vi "playsound.vi"(11 "Sound File Path":path=path "../support/sample.wav") -> ()   [LabVIEW 2014]
uses:
  <vilib>/sound2/lvsound2.llb/Sampling Mode.ctl
  <vilib>/sound2/lvsound2.llb/Sound File Info (path).vi
  <vilib>/sound2/lvsound2.llb/Sound File Read Open.vi
  <vilib>/sound2/lvsound2.llb/Sound File Read (DBL).vi
  <vilib>/sound2/lvsound2.llb/Sound Output Write (DBL).vi
panel:
  in  "Number of Samples/Iteration":i32=2500
  in  "Device ID":u32
  in  "Stop":bool
  out "Current Iteration":i32
  out "Current Data":waveform(dbl)[](graph)
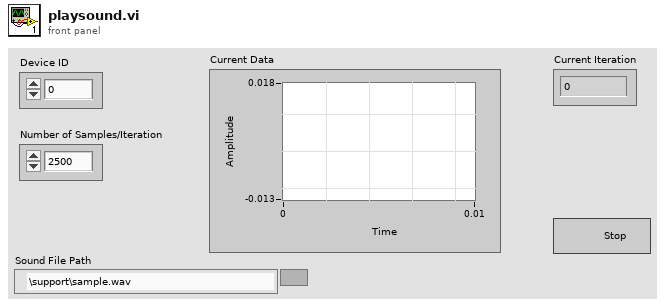
[diagram p1: front panel]
types:
  T1 = typedef "Sampling Mode.ctl" = i32
  T2 = typedef "Sound Data Format.ctl" = cluster{"sample rate (S/s)":dbl, "number of channels":i32, "bits per sample":i32}
  T3 = typedef "Sound File Refnum.ctl" = refnum<file>
  T4 = typedef "Sound Output Task ID.ctl" = u32
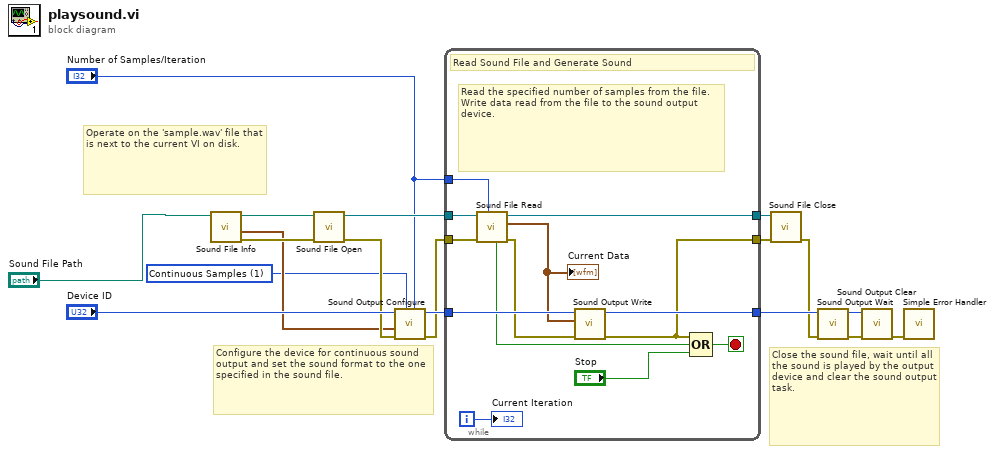
[diagram p0: block diagram]
diagram:
  w3 = T1 1 items=["Finite Samples", "Continuous Samples"] ("sample mode")
  # "Operate on the 'sample.wav' file that is next to the current VI on disk."
  # "Close the sound file, wait until all the sound is played by the output device and clear the sound output task."
  # "Configure the device for continuous sound output and set the sound format to the one specified in the sound file."
  n1 = call-poly <vilib>:"Sound File Info.vi"("path"="Sound File Path") -> ("error out"=w13:errorcluster, "sound format"=w5:T2, "path out"=w6:path)  [unwired: 7 in, 1 out]
  n2 = call-poly <vilib>:"Sound File Open.vi"("error in (no error)"=w13, "path"=w6) -> ("error out"=w12:errorcluster, "sound file refnum"=w14:T3)  [unwired: 8 in]
  n3 = call <vilib>:"Sound Output Configure.vi"("number of samples/ch"="Number of Samples/Iteration", "sample mode"=w3, "error in (no error)"=w12, "sound format"=w5, "device ID"="Device ID") -> ("error out"=w11:errorcluster, "task ID"=w18:T4)  [unwired: 5 in]
  n4 = while {
    tunnel: "Number of Samples/Iteration" -> [w21]
    tunnel: w14 -> [w29]
    tunnel: [w27] -> w16
    tunnel: w11 -> [w30]
    tunnel: [w20] -> w15
    tunnel: w18 -> [w26]
    tunnel: [w31] -> w9
    i -> [w28]
    stop <- w22 stop-if-true
    # "Read the specified number of samples from the file. Write data read from the file to the sound output device."
    # "Read Sound File and Generate Sound"
    n5 = call-poly <vilib>:"Sound File Read.vi"("number of samples/ch (-1: all)"=w21, "error in (no error)"=w30, "sound file refnum"=w29) -> ("error out"=w25:errorcluster, "data"=w19:waveform(dbl)[], "sound file refnum out"=w27:T3, "end of file?"=w23:bool)  [unwired: 4 in, 1 out]
    "Current Data" <- w19
    n6 = call-poly <vilib>:"Sound Output Write.vi"("error in (no error)"=w25, "data"=w19, "task ID"=w26) -> ("error out"=w20:errorcluster, "task ID out"=w31:T4)  [unwired: 7 in]
    n7 = Compound Arithmetic op=OR(w20, w23, "Stop") -> (w22:bool)
    "Current Iteration" <- w28
  }
  n8 = call <vilib>:"Sound File Close.vi"("error in (no error)"=w15, "sound file refnum"=w16) -> ("error out"=w8:errorcluster)  [unwired: 9 in]
  n9 = call <vilib>:"Sound Output Wait.vi"("error in (no error)"=w8, "task ID"=w9) -> ("error out"=w7:errorcluster, "task ID out"=w10:T4)  [unwired: 8 in]
  n10 = call <vilib>:"Sound Output Clear.vi"("error in (no error)"=w7, "task ID"=w10) -> ("error out"=w2:errorcluster)  [unwired: 9 in]
  n11 = call <vilib>:"Simple Error Handler.vi"("error in (no error)"=w2) -> ()  [unwired: 4 in, 5 out]
